vi "FPGA.vi"() -> ()   [LabVIEW 2021]
uses:
  <vilib>/rvi/Emulation/niFpgaGetClockAttributes.vi
  <vilib>/rvi/Emulation/niFpgaSctlEmulationGetInTimedLoop.vi
  <vilib>/rvi/Emulation/niFpgaEmulationReportErrorSimple.vi
  <vilib>/rvi/eio/common/nirviEmuTemplateMethod_errors.vi
  <vilib>/rvi/interface/RandomDataEmulation/niFpgaRandomDataHandleErrors.vi
  <vilib>/rvi/Emulation/niFpgaCriticalErrorInLSC.vi
  <vilib>/eio/EIONode/EIONode.xnode
  <vilib>/rvi/DataTransferAndStorage/Container/XNode/niFpgaContainer.xnode
  <vilib>/rvi/interface/RandomDataEmulation/nirviRandomDataFpgaReadWriteTemplate.vi
panel:
  out "to RT overflow":bool
  out "From RT underflow?":bool
  in  "loop time(uSec)":u32 caption="Count(uSec)"
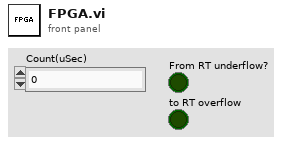
[diagram p1: front panel]
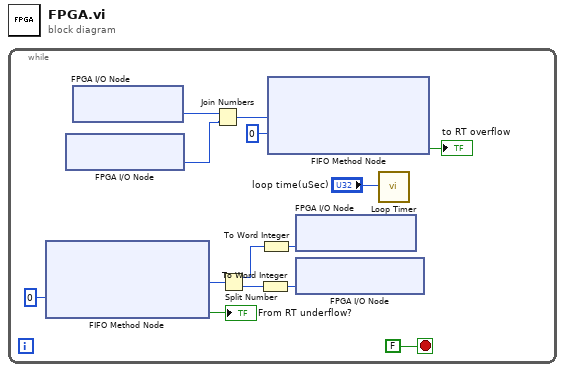
[diagram p0: block diagram]
diagram:
  n1 = while {
    stop <- FALSE stop-if-true
    n2 = xnode ("FIFO Method Node")("Timeout"=0) -> ("Element"=w5:u32, "Timed Out?"=→"From RT underflow?":bool)  [unwired: 1 in, 1 out]
    n3 = xnode "FPGA I/O Node"() -> ("AudioIn/Right"=w8:i16)  [unwired: 1 in, 1 out]
    n4 = xnode "FPGA I/O Node"() -> ("AudioIn/Left"=w9:i16)  [unwired: 1 in, 1 out]
    n5 = Join Numbers(hi=w9, lo=w8) -> ((hi.lo)=w6:u32)
    n6 = Split Number(x=w5) -> (hi(x)=w10:u16, lo(x)=w11:u16)
    n7 = To Word Integer(number=w11) -> (16bit integer=w12:i16)
    n8 = To Word Integer(number=w10) -> (16bit integer=w13:i16)
    n9 = xnode ("FIFO Method Node")("Element"=w6, "Timeout"=0) -> ("Timed Out?"=→"to RT overflow":bool)  [unwired: 1 in, 1 out]
    n10 = xnode "FPGA I/O Node"("AudioOut/Left"=w13) -> ()  [unwired: 1 in, 1 out]
    n11 = xnode "FPGA I/O Node"("AudioOut/Right"=w12) -> ()  [unwired: 1 in, 1 out]
    n12 = call "Loop Timer"("Count(uSec)"="loop time(uSec)") -> ()  [unwired: 1 out]
  }
